vi "WfmMain.vi"() -> ()   [LabVIEW 2012]
doc: "使用该模板构建简单状态机设计模式。各状态执行代码并决定转移状态。"
uses:
  controls/WfmState.ctl
  controls/WfmData.ctl
panel:
  out "波形图":dbl[](graph)
  in  "记录至文件":bool
  in  "采集波形":bool
  in  "停止按钮":bool
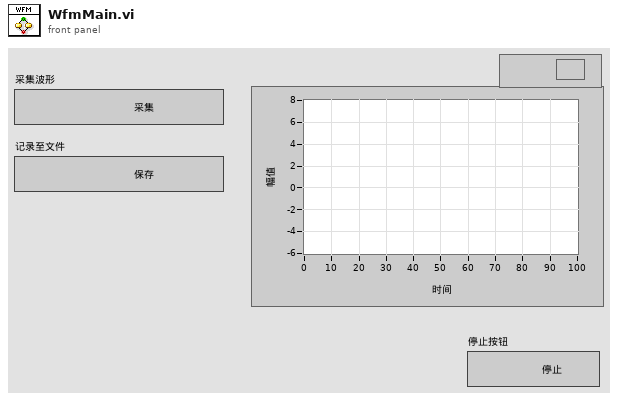
[diagram p1: front panel]
types:
  T1 = typedef "WfmData.ctl" = cluster{"数组":dbl[]}
  T2 = typedef "WfmState.ctl" = enum16{"初始化", "等待事件", "采集波形", "记录至文件", "停止"}
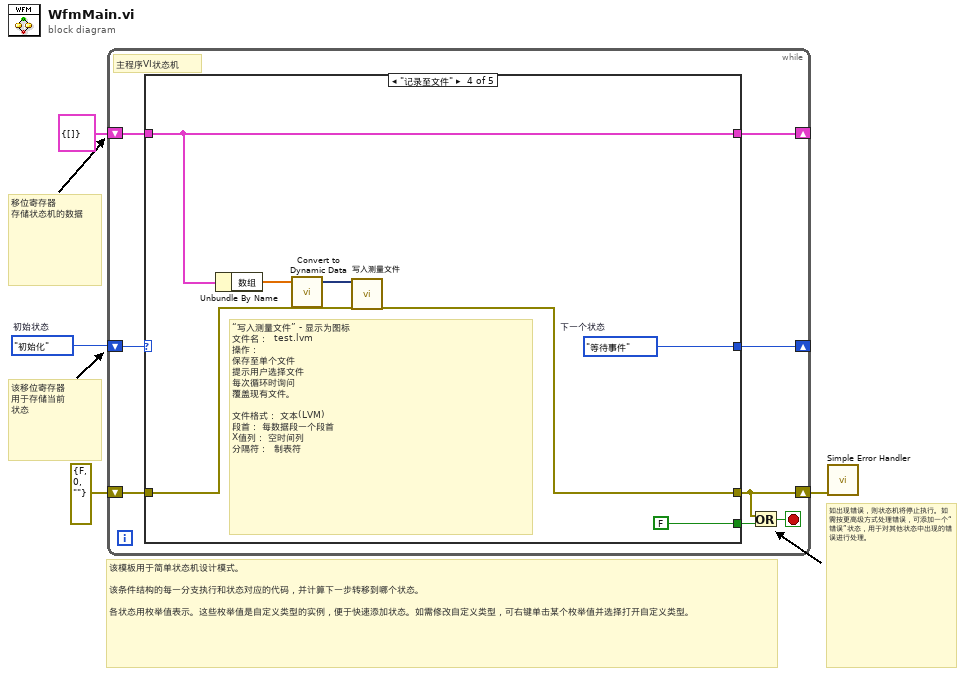
[diagram p0: block diagram]
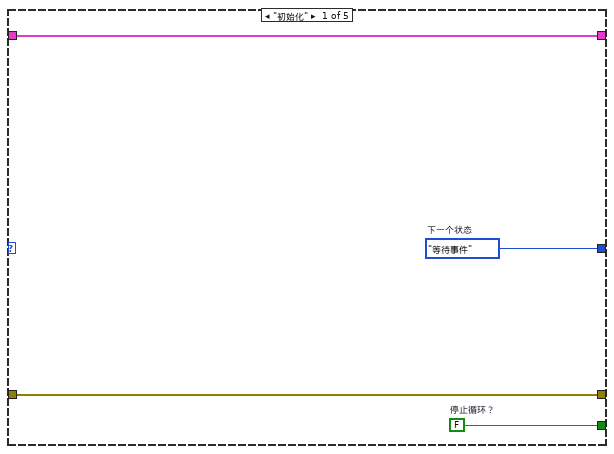
[diagram p2: hidden frame]
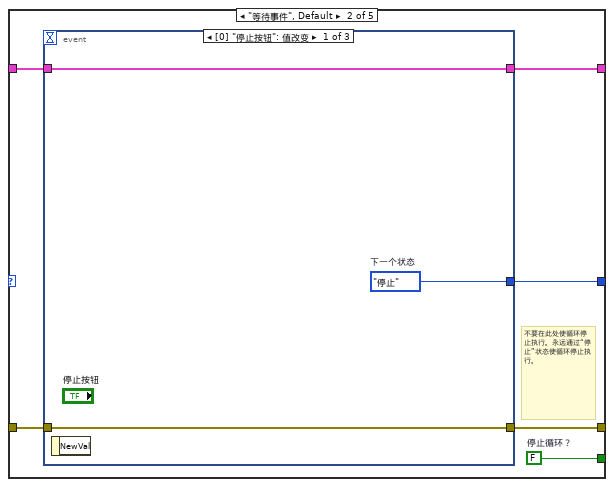
[diagram p3: hidden frame]
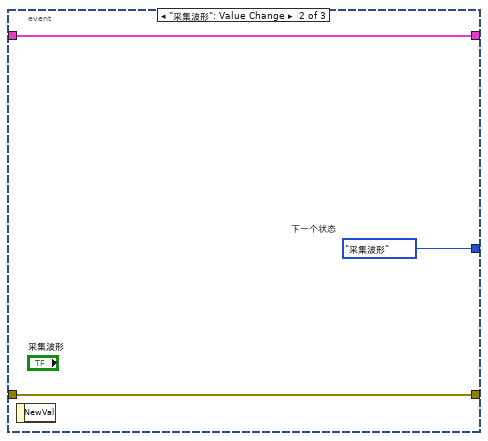
[diagram p4: hidden frame]
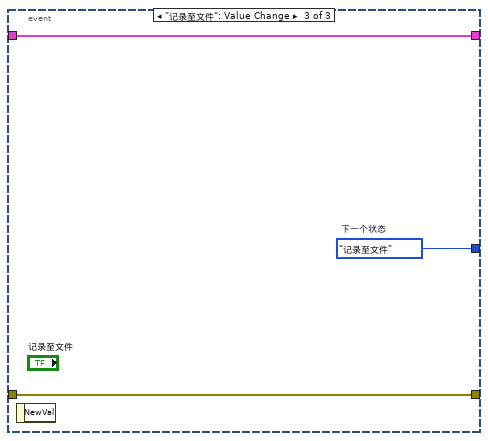
[diagram p5: hidden frame]
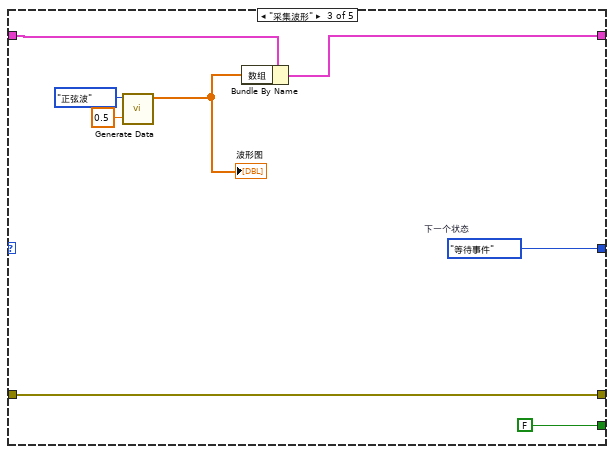
[diagram p6: hidden frame]
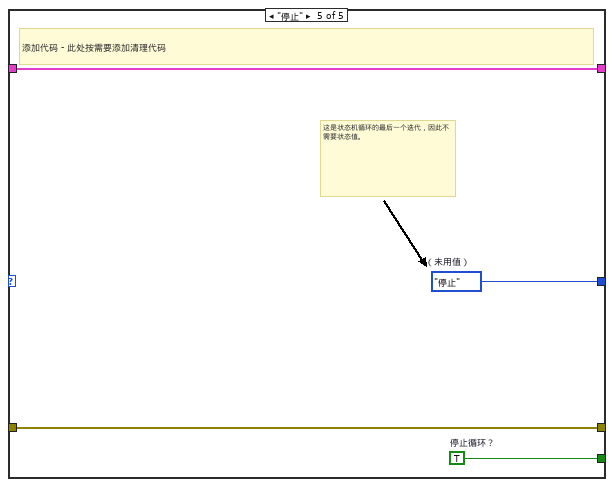
[diagram p7: hidden frame]
diagram:
  w4 = WfmState."初始化"  # 初始状态
  # "如出现错误，则状态机将停止执行。如需按更高级方式处理错误，可添加一个“错误”状态，用于对其他状态中出现的错误进行处理。"
  # "移位寄存器\n存储状态机的数据"
  # "该模板用于简单状态机设计模式。\n\n该条件结构的每一分支执行和状态对应的代码，并计算下一步转移到哪个状态。\n\n各状态用枚举值表示。这些枚举值是自定义类型的实例，便于快速添加状态。如需修改自定义类型，可右键单击某个枚举值并选择打开自定义类型。"
  # "该移位寄存器\n用于存储当前\n状态"
  n1 = while {
    shift-right: [w11] -> _
    shift-left: w4 -> [w12]
    shift-right: [w9] -> _
    shift-left: T1 {"数组"=[]} ("数据") -> [w10]
    shift-right: [w5] -> w1
    shift-left: cluster{"状态":bool, "代码":i32, "源":string} {"状态"=FALSE, "代码"=0, "源"=""} ("错误常量") -> [w8]
    stop <- w6 stop-if-true
    # "主程序VI状态机"
    n2 = case shown="\"记录至文件\"" w12 {
      tunnel: [w16 w22 w39 w46 w50] -> w11
      tunnel: [w15 w21 FALSE ("停止循环？") FALSE ("停止循环？") w48] -> w7
      tunnel: w10 -> [w13 w20 w37 w44 w49]
      tunnel: [w13 w19 w36 w44 w49] -> w9
      tunnel: w8 -> [w14 w18 w34 w41 w47]
      tunnel: [w14 w17 w34 w40 w47] -> w5
      frame "初始化" {
        w15 = FALSE  # 停止循环？
        w16 = WfmState."等待事件"  # 下一个状态
      }
      frame "等待事件", Default {
        w21 = FALSE  # 停止循环？
        # "不要在此处使循环停止执行。永远通过“停止”状态使循环停止执行。"
        n3 = event shown="[0] \"停止按钮\": 值改变" {
          selector: _ -> [_ _ _]
          dyn-events: _ -> [_ _ _]
          timeout: _ -> [_ _ _]
          tunnel: [w25 w28 w31] -> w22
          tunnel: w20 -> [w24 w26 w29]
          tunnel: [w24 w26 w29] -> w19
          tunnel: w18 -> [w23 w27 w30]
          tunnel: [w23 w27 w30] -> w17
          event "停止按钮": Value Change {
            w25 = WfmState."停止"  # 下一个状态
            n4 = event-data ("事件数据节点")() -> ()  [unwired: 1 in, 1 out]
          }
          event "采集波形": Value Change {
            w28 = WfmState."采集波形"  # 下一个状态
            n5 = event-data ("事件数据节点")() -> ()  [unwired: 1 in, 1 out]
          }
          event "记录至文件": Value Change {
            w31 = WfmState."记录至文件"  # 下一个状态
            n6 = event-data ("事件数据节点")() -> ()  [unwired: 1 in, 1 out]
          }
        }
      }
      frame "采集波形" {
        w39 = WfmState."等待事件"  # 下一个状态
        n7 = call "Generate Data.vi"("噪声(rms)"=0.5, "信号"=enum16{"均匀白噪声", "均匀+均匀", "高斯白噪声", "正弦波", "方波"}."正弦波") -> ("Y"=w35:dbl[])  [unwired: 8 in, 1 out]
        "波形图" <- w35
        n8 = Bundle By Name ("按名称捆绑")(cluster=w37, "数组"=w35) -> (w36:T1)
      }
      frame "记录至文件" {
        w46 = WfmState."等待事件"  # 下一个状态
        # "“写入测量文件” - 显示为图标\n文件名：  test.lvm\n操作：\n保存至单个文件\n提示用户选择文件\n每次循环时询问\n覆盖现有文件。\n\n文件格式： 文本(LVM)\n段首： 每数据段一个段首\nX值列： 空时间列\n分隔符：  制表符"
        n9 = Unbundle By Name ("按名称解除捆绑")(w44) -> ("数组"=w43:dbl[])
        n10 = call "Convert to Dynamic Data"("Array"=w43) -> ("Dynamic Data Type"=w42:dynamicdata)  [unwired: 3 in]
        n11 = call "写入测量文件"("Signals"=w42, "error in (no error)"=w41) -> ("error out"=w40:errorcluster)  [unwired: 15 in, 2 out]
      }
      frame "停止" {
        w48 = TRUE  # 停止循环？
        w50 = WfmState."停止"  # （未用值）
        # "添加代码 - 此处按需要添加清理代码"
        # "这是状态机循环的最后一个迭代，因此不需要状态值。"
      }
    }
    n12 = Or ("或")(x=w5, y=w7) -> (x .or. y?=w6:bool)
  }
  n13 = call <vilib>:"Simple Error Handler.vi"("error in (no error)"=w1) -> ()  [unwired: 4 in, 5 out]
